vi "Configure Interpolation [I].vi"(8 "error in (no error)":errorcluster, 10 "interpolation":i32(ring)=1 items=["No Interpolation"=1, "sin(x)/x"=2, "Linear Interpolation"=3], 11 "CS++Scope":refnum<class "CS++Scope.lvclass">) -> (0 "error out":errorcluster, 3 "CS++Scope out":refnum<class "CS++Scope.lvclass">)   [LabVIEW 2015, in "CS++Scope.lvlib" / "CS++Scope.lvclass"]
doc: "This VI configures the interpolation method the oscilloscope uses when it cannot sample a voltage for a point in the waveform record. \n\nNotes:\n\n(1) This VI is part of the miscellaneous [*] extension group."
uses:
  CS++Scope.lvclass
  CSPP_Core/Classes/CS++ProcessVariables/ProcessVariable/PV.lvclass
  PV-Enum.ctl
  CSPP_Core/Classes/CS++ProcessVariables/ProcessVariable/PV.lvclass/PV.ctl
  CS++Scope.lvclass/CS++Scope.ctl
  CSPP_Core/Classes/CS++ProcessVariables/ProcessVariable/Write Data.vi
  CSPP_Core/Classes/CS++ProcessVariables/ProcessVariable/Write Timestamp.vi
  CSPP_Core/Classes/CS++ProcessVariables/ProcessVariable/Write Quality.vi
  CSPP_Core/Classes/CS++ProcessVariables/ProcessVariable/Write status.vi
  CSPP_Core/Classes/CS++ProcessVariables/PVConnection/PVConnection.lvclass
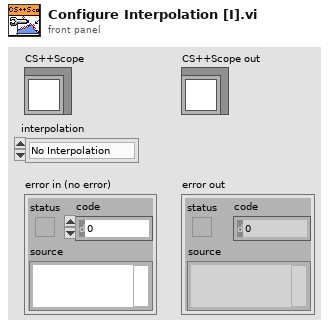
[diagram p1: front panel]
types:
  T1 = typedef "CS++Scope.lvlib/CS++Scope.lvclass/PV-Enum.ctl" = enum16{"ActualSampleRate", "TimePerRecord", "AcquisitionStartTime", "TriggerLevel", "GlitchWidth", "LowReference", "MidReference", "HighReference", "RuntLowThreshold", "RuntHighThreshold", "TriggerHoldoff", "WidthLowThreshold", "WidthHighThreshold", "AcquisitionStatus", "ActualRecordLength", "ActualSampleMode", "ACLineTriggerSlope", "MinRecordLength", "AcquisitionType", "TriggerSlope", "GlitchCondition", "GlitchPolarity", "InterpolationMethod", "NumberOfAverages", "NumberOfEnvelopes", "TriggerType", "TriggerCoupling", "TriggerModifier", "TVLineNumber", "TVEvent", "TVTriggerPolarity", "TVSignalFormat", "WidthCondition", "WidthPolarity", "MeasurementDone", "ContinousAcquisition", "TriggerSource", "Waveform", "ActualTimeIncrement"}
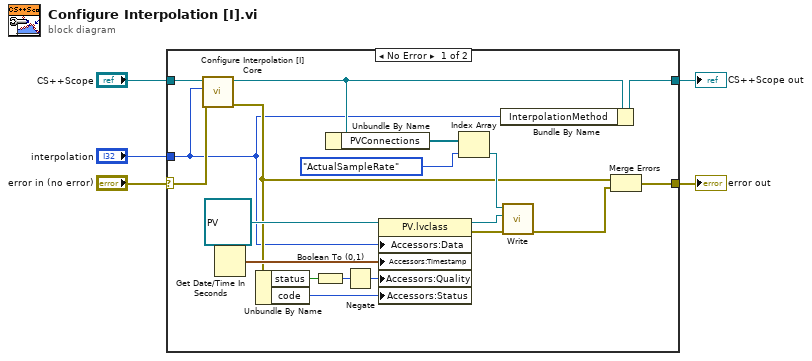
[diagram p0: block diagram]
diagram:
  n1 = case shown="No Error" "error in (no error)" {
    selector: "error in (no error)" -> [w8 w26]
    tunnel: [w7 w26] -> w4
    tunnel: [w9 w25] -> w2
    tunnel: "CS++Scope" -> [w10 w25]
    tunnel: "interpolation" -> [w6 _]
    frame No Error {
      n2 = call-dynamic "Configure Interpolation [I] Core.vi"("error in (no error)"=w8, "interpolation"=w6, "CS++Scope"=w10) -> ("error out"=w12:errorcluster, "CS++Scope out"=w24:refnum<class "CS++Scope.lvclass">)  [unwired: 7 in]
      n3 = Get Date/Time In Seconds() -> (seconds since 1Jan1904=w18:timestamp)
      n4 = Unbundle By Name(w12) -> ("status"=w21:bool, "code"=w22:i32)
      n5 = Boolean To (0,1)(Boolean=w21) -> (0, 1=w20:i16)
      n6 = Unbundle By Name(w24) -> ("PVConnections"=w15:refnum<class "PVConnection.lvclass">[])
      n7 = Negate(x=w20) -> (-x=w19:i16)
      n8 = property class="PV.lvclass"(reference=refnum<class "PV.lvclass"> refnum ("CS++ProcessVariables.lvlib:PV.lvclass"), "Accessors:Data"=w6, "Accessors:Timestamp"=w18, "Accessors:Quality"=w19, "Accessors:Status"=w22) -> (reference out=w17:refnum<class "PV.lvclass">, error out=w16:errorcluster)  [unwired: 1 in]
      n9 = Index Array(array=w15, index=PV-Enum."ActualSampleRate" ("PV-Enum")) -> (element=w13:refnum<class "PVConnection.lvclass">)
      n10 = Bundle By Name(cluster=w24, "InterpolationMethod"=w6) -> (w9:refnum<class "CS++Scope.lvclass">)
      n11 = call "Write.vi"("error in (no error)"=w16, "PV"=w17, "PVConnection in"=w13) -> ("error out"=w11:errorcluster)  [unwired: 7 in, 1 out]
      n12 = Merge Errors(w12, w11) -> (w7:errorcluster)
    }
    frame Error {
    }
  }
  "error out" <- w4
  "CS++Scope out" <- w2
